vi "Tetra_TX-ATTEN_Setup.vi"() -> (0 "error out":errorcluster, 2 "Status":string="Skipping Setup of Power Supply\rDone !!!\rDONE!!\n\nSetting up PNA...\rRecalling PNA Setup:  Z:\\State Files\\TEST2.csa\rDONE!!!\rSkipping Spectrum Analyzer!!!\rSkipping Setting Up Temperature...\rSetup Complete !!!")   [LabVIEW 2018]
uses:
  <vilib>/Utility/error.llb/DialogType.ctl
  Tetra_Globals.vi
  Initialize References/Sequence Globals.vi
  Infrastructure/Test Parameter Globals_1.0.0.vi
  Initialize References/Station References Global.vi
  Infrastructure/Test Result File Name Global.vi
  <vilib>/Utility/file.llb/Read Delimited Spreadsheet (string).vi
  <vilib>/Utility/file.llb/Write Delimited Spreadsheet (string).vi
  Instruments/PNA/lib functions/Agilent ENA Series.lvlib
  Instruments/Agilent N5232A PNA-L/Labview Driver/Keysight PNA Series/Keysight PNA Series.lvlib
panel:
  in  "ess_error":errorcluster
  in  "Tab Control":T1(tab)
  in  "Setup Chip (T)":bool=TRUE
  in  "Setup Power Supply (T)":bool=TRUE
  in  "Setup PNA (T)":bool=TRUE
  in  "Kill Teraterm":bool=TRUE
  in  "Setup Gantry(t)":bool=TRUE
  in  "Setup EXA(t)":bool=TRUE
  out "Success":bool
  out "MODE":bool
  out "COM PORT":string="COM4"
  out "RevC(t)":bool
  out "RBW":string="3000"
  out "Avgs":u32=4
  out "SPAN":dbl=0.1
  out "REF_LVL":dbl=10.0
  out "PS1-1(V)":dbl=18.75
  out "PS1-1(A)":dbl=1.0
  out "PS1-2(V)":dbl=5.0
  out "PS1-2(A)":dbl=1.0
  out "Use PS1-2":bool=TRUE
  out "Use PS1-1":bool=TRUE
  out "EXA State File":string="Z:\\State Files\\State_0000.state"
  out "cmd;":string
  out "TEMP":dbl=25.0
  out "TEMP?(t)":bool
  out "RF_FREQ":dbl=20.0
  out "f_ref":dbl=10.0
  out "REF_POWER":dbl=7.5
  out "Soak Time (s)":dbl=10.0 caption="Delay Time (s)"
  out "Ant":i16
  out "Gantry-Z":dbl
  out "GET_DET":bool
  out "OUT_CAL_PATH":path=path "C:/RageATE/Automated Tests/Tetra WAM/DVT/Cal Files/OUTPUT_CAL_080321-1118.csv"
  out "HORN_CAL_PATH":path
  out "REF_CAL_PATH":path
  out "git log":string="#RageATE gitlog: commit 9dda47de5732cf8fa6a9554b7d9ab91f125b5971\n#RageATE gitlog: Author: rick-rage <rick@ragesystems.com>\n#RageATE gitlog: Date:   Mon Aug 2 15:21:18 2021 -0400\n#RageATE gitlog: This Computer Name : CRANES\r\n\r\n"
  out "PNA State File":string="Z:\\State Files\\TEST2.csa"
  out "Text":refnum<vi>
  out "OUT_CAL_PATH(str)":string
  out "Pmic_FwRev":string
  out "i_mon":string
  out "rev":string="rdiv\r\n0)  sw3p6:   195 mA  3616 mV\r\n1)  sw5p5:    89 mA  5472 mV\r\n2) sw2p8a:   315 mA  2784 mV\r\n3) sw2p8b:   349 mA  2768 mV\r\n4)  sw2p4:  1458 mA  2288 mV\r\n5)  sw1p4:  1047 mA  1304 mV\r\n>"
  out "snic":string="#Family: 0x2D\n#Serial: 0x000036092740\r\n"
  in  "error in (no error)":errorcluster
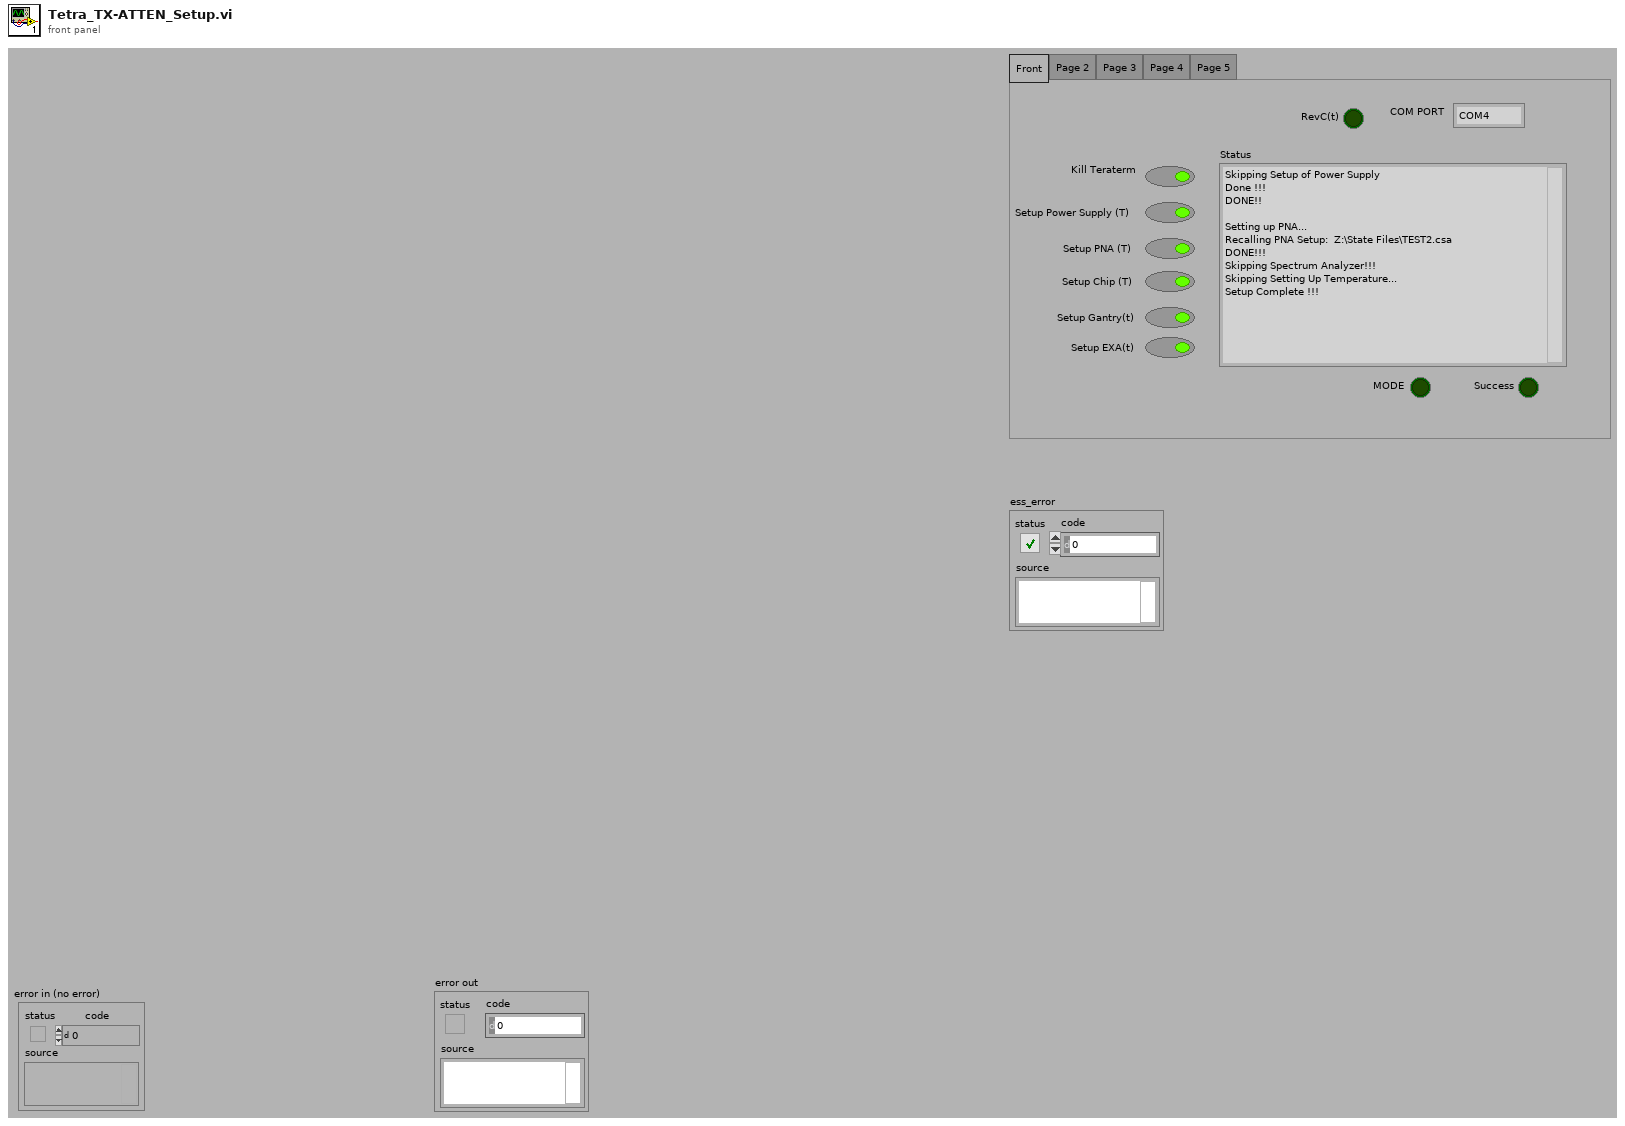
[diagram p1: front panel]
types:
  T1 = enum32{"Front", "Page 2", "Page 3", "Page 4", "Page 5"}
  T2 = typedef "DialogType.ctl" = u16
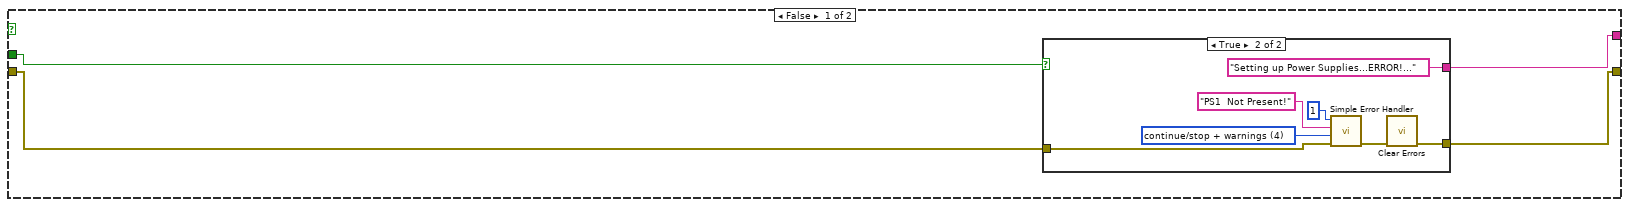
[diagram p8: hidden frame]
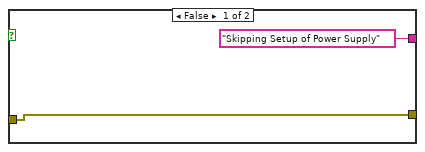
[diagram p9: hidden frame]
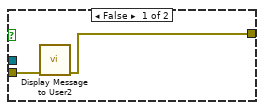
[diagram p11: hidden frame]
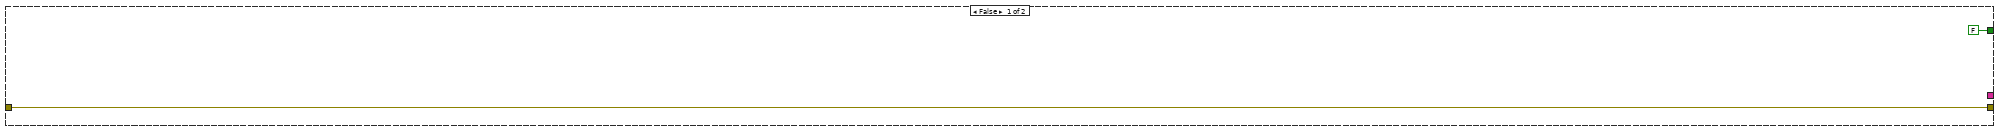
[diagram p12: hidden frame]
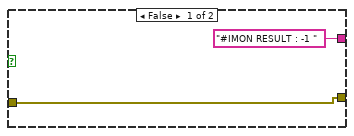
[diagram p13: hidden frame]
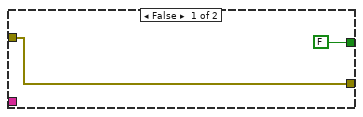
[diagram p14: hidden frame]
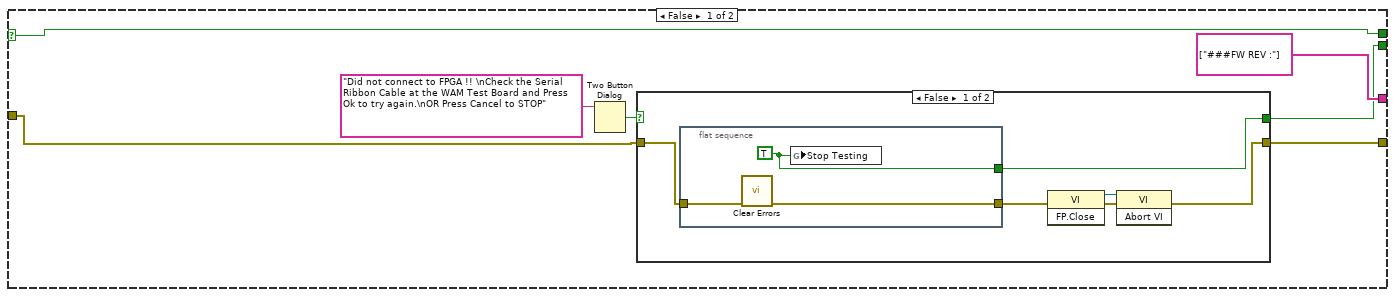
[diagram p15: hidden frame]
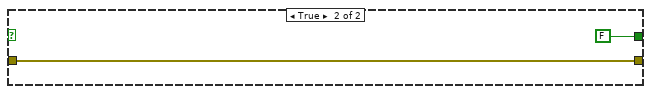
[diagram p16: hidden frame]
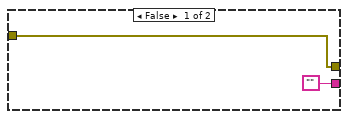
[diagram p17: hidden frame]
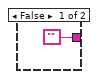
[diagram p19: hidden frame]
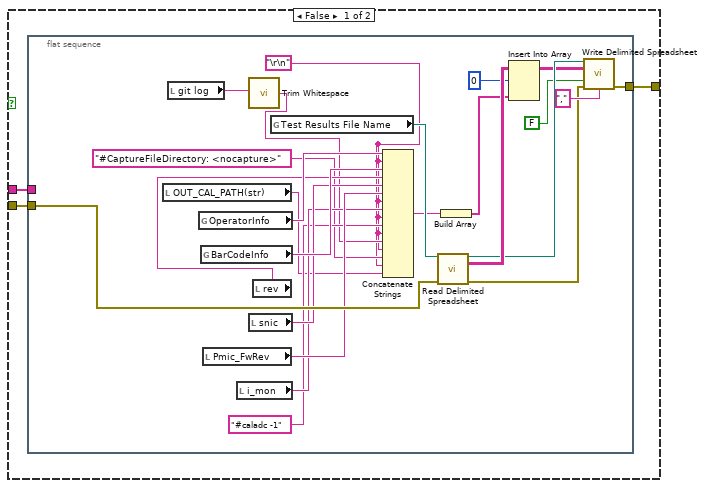
[diagram p20: hidden frame]
diagram:
  n1 = flat-sequence {
    tunnel: [w52] -> w6
    tunnel: [w51] -> w5
    tunnel: w6 -> [w111]
    tunnel: w5 -> [w110]
    tunnel: [w251] -> w8
    tunnel: [w249] -> w7
    tunnel: w8 -> [w441]
    tunnel: w7 -> [w439]
    tunnel: [w435] -> w3
    tunnel: [w520] -> w4
    tunnel: w3 -> [w523]
    tunnel: w4 -> [w591]
    tunnel: [w586] -> w10
    tunnel: [w590] -> w9
    tunnel: w10 -> [w629]
    tunnel: w9 -> [w632]
    tunnel: [w621] -> w1
    frame #0 {
      # "Automated Tests\\Tetra WAM\\PRODUCTION\\Test Benches"
      # "Kill TeraTerm"
      n2 = flat-sequence {
        tunnel: [w38] -> w16
        frame #0 {
          w35 = 1 items=["INPUT", "OUTPUT"] ("line index")
          (unwired) path "C:/RageATE/Automated Tests/Tetra WAM/PRODUCTION/Test Benches" ("base path")
          n3 = global read "Sequence Globals.vi" "DevSupportPath"() -> (w27:path)
          n4 = Strip Path(path=w27) -> (stripped path=w26:path)  [unwired: 1 out]
          n5 = global read "Sequence Globals.vi" "AppSupportPath"() -> (w32:path)
          n6 = Build Path(base path=w26, name or relative path=path "Automated Tests/Tetra WAM/PRODUCTION/Test Benches" ("base path")) -> (appended path=w24:path)
          n7 = global read "Sequence Globals.vi" "IsRuntime?"() -> (w23:bool)
          n8 = global read "Tetra_Globals.vi" "TestBench_ID"() -> (w28:string)
          n9 = Build Path(base path=w24, name or relative path=w28) -> (appended path=w37:path)
          n10 = Concatenate Strings(w28, " Calibration Files" ("name or relative path")) -> (w29:string)
          n11 = Build Path(base path=w37, name or relative path=w29) -> (appended path=w34:path)
          n12 = Select(t=w32, s=w23, f=w34) -> (s? t:f=w33:path)
          n13 = call "FindMostRecentCalFile.vi"("DIR_IN"=w33, "Test Bench (for filename match)"=w28, "line index"=w35, "IsRuntime?"=w23) -> ("Success?(t)"=w30:bool, "cal_path_out"=w31:path)  [unwired: 9 in, 1 out]
          n14 = case shown="False" w30 {
            tunnel: [path "" ("appended path") w41] -> w38
            tunnel: w31 -> [_ w41]
            frame False {
              n15 = Two Button Dialog(message="There Are No OUTPUT cal files") -> ()  [unwired: 2 in, 1 out]
            }
            frame True {
            }
          }
        }
      }
      n16 = global read "Sequence Globals.vi" "RageATE_Gitlog"() -> (→"git log":string)
      n17 = global read "Tetra_Globals.vi" "RevC(t)"() -> (→"RevC(t)":bool)
      n18 = case shown="True" "Kill Teraterm" {
        tunnel: "error in (no error)" -> [w42 w44]
        tunnel: [w42 w43] -> w18
        tunnel: "taskkill /f /im ttermpro.exe" ("command line") -> [_ w46]
        frame False {
        }
        frame True {
          n19 = call <vilib>:"Clear Errors.vi"("error in (no error)"=w44) -> ("error out"=w45:errorcluster)  [unwired: 5 in, 1 out]
          n20 = call <vilib>:"System Exec.vi"("error in (no error)"=w45, "command line"=w46) -> ("error out"=w47:errorcluster)  [unwired: 6 in, 3 out]
          n21 = call "Time Delay2"("error in (no error)"=w47) -> ("error out"=w43:errorcluster)  [unwired: 10 in]
        }
      }
      n22 = property on="Status" class="Str"(error in=w18) -> (error out=w17:errorcluster, "Text"=→"Text":refnum<vi>)  [unwired: 1 in, 1 out]
      n23 = local write "error in (no error)"(w17) -> ()
      n24 = Path To String(path=w16) -> (string=w15:string)
      n25 = Concatenate Strings("#Cal_Path: " ("string"), w15) -> (→"OUT_CAL_PATH(str)":string)
      "OUT_CAL_PATH" <- w16
    }
    frame #1 {
      # "TEMP\nPS1-1_V\nRF_FREQ_OUT\nTX_PORT\nTX_FILT\nADAR_ATT\nPSA_ATT\nREF_POWER"
      n26 = local write "Success"(FALSE ("Success")) -> ()
      n27 = local write "Setup PNA (T)"("Setup PNA (T)") -> ()
      n28 = local write "Setup EXA(t)"("Setup EXA(t)") -> ()
      n29 = local write "Setup Gantry(t)"("Setup Gantry(t)") -> ()
      n30 = local write "Setup Chip (T)"("Setup Chip (T)") -> ()
      n31 = local write "Setup Power Supply (T)"("Setup Power Supply (T)") -> ()
      n32 = global read "Test Parameter Globals_1.0.0.vi" "Input Constants Out"() -> (w52:string[])
      n33 = global read "Test Parameter Globals_1.0.0.vi" "Test Parameters"() -> (w51:string[][])
      "Status" <- ""
    }
    frame #2 {
      w107 = 0 ("disabled index (col)")
      w96 = 11  # index
      n34 = Index Array(array=w110, index (row) #1=0 ("disabled index (row)"), index (col) #1=w107, index (row) #2=7 ("disabled index (row)"), index (col) #2=w107, index (row) #3=2 ("disabled index (row)"), index (col) #3=w107) -> (element #1=w105:string, element #2=w103:string, element #3=w101:string)
      n35 = Index Array(array=w111, index #6=w96) -> (element #1=w119:string, element #2=w112:string, element #3=w73:string, element #4=w100:string, element #5=w80:string, element #6=w95:string, element #7=w81:string, element #8=w97:string, element #9=→"PNA State File":string, element #10=→"EXA State File":string, element #11=→"RBW":string, element #12=w88:string, element #13=w85:string, element #14=w83:string, element #15=w57:string, element #16=w65:string)  [unwired: 15 in]
      "cmd;" <- w81
      n36 = global write "Tetra_Globals.vi" "cmd;"(w81) -> ()
      n37 = call "StringToNumberControlWithBool.vi"("String In"=w103) -> ("Number Out"=→"REF_POWER":dbl)  [unwired: 7 in, 1 out]
      n38 = call "TempControlWithBool.vi"("INPUT"=w105) -> ("out"=→"TEMP":dbl, "Valid(t)"=→"TEMP?(t)":bool)  [unwired: 6 in, 1 out]
      n39 = call "StringToNumberControlWithBool.vi"("String In"=w101) -> ("Number Out"=w93:dbl)  [unwired: 7 in, 1 out]
      "RF_FREQ" <- w93
      n40 = global read "Tetra_Globals.vi" "comport"() -> (w71:refnum<visa-resource-name>)
      n41 = Empty String/Path?(string/path=w73) -> (empty?=w74:bool)
      n42 = global read "Sequence Globals.vi" "AppSupportPath"() -> (w68:path)
      n43 = call "StringToNumberControlWithBool.vi"("String In"=w100) -> ("NOT = 0"=→"MODE":bool)  [unwired: 7 in, 1 out]
      n44 = call "StringToNumberControlWithBool.vi"("String In"=w95) -> ("NOT = 0"=→"GET_DET":bool)  [unwired: 7 in, 1 out]
      n45 = call "StringToNumberControlWithBool.vi"("String In"=w97) -> ("Number Out"=→"Soak Time (s)":dbl)  [unwired: 7 in, 1 out]
      n46 = call "StringToNumberControlWithBool.vi"("String In"=w88) -> ("Number Out"=→"Avgs":dbl)  [unwired: 7 in, 1 out]
      n47 = call "StringToNumberControlWithBool.vi"("String In"=w85) -> ("Number Out"=→"REF_LVL":dbl)  [unwired: 7 in, 1 out]
      n48 = call "StringToNumberControlWithBool.vi"("String In"=w83) -> ("Number Out"=→"SPAN":dbl)  [unwired: 7 in, 1 out]
      n49 = global read "Sequence Globals.vi" "IsRuntime?"() -> (w70:bool)
      n50 = String To Path(string=w57) -> (path=→"REF_CAL_PATH":path)
      n51 = Divide(x=w93, y=2.0) -> (x/y=→"f_ref":dbl)
      n52 = Match Pattern(string=w119, regular expression=";") -> (before substring=w126:string, after substring=w125:string)  [unwired: 1 in, 2 out]
      n53 = Match Pattern(string=w112, regular expression=";") -> (before substring=w117:string, after substring=w116:string)  [unwired: 1 in, 2 out]
      n54 = Match Pattern(string=w80, regular expression=";") -> (before substring=w78:string, after substring=w77:string)  [unwired: 1 in, 2 out]
      n55 = Select(t=w71, s=w74, f=w73) -> (s? t:f=→"COM PORT":refnum<visa-resource-name>)
      n56 = call "StringToNumberControlWithBool.vi"("String In"=w125) -> ("Number Out"=→"PS1-1(A)":dbl)  [unwired: 7 in, 1 out]
      n57 = call "StringToNumberControlWithBool.vi"("String In"=w116) -> ("Number Out"=→"PS1-2(A)":dbl)  [unwired: 7 in, 1 out]
      n58 = call "StringToNumberControlWithBool.vi"("String In"=w126) -> ("Number Out"=→"PS1-1(V)":dbl, "NOT = 0"=→"Use PS1-1":bool)  [unwired: 7 in]
      n59 = call "StringToNumberControlWithBool.vi"("String In"=w117) -> ("Number Out"=→"PS1-2(V)":dbl, "NOT = 0"=→"Use PS1-2":bool)  [unwired: 7 in]
      n60 = call "StringToNumberControlWithBool.vi"("String In"=w78) -> ("Number Out"=→"Ant":dbl, "NOT = 0"=w86:bool)  [unwired: 7 in]
      n61 = call "StringToNumberControlWithBool.vi"("String In"=w77) -> ("Number Out"=w76:dbl)  [unwired: 7 in, 1 out]
      "Gantry-Z" <- w76
      n62 = global write "Tetra_Globals.vi" "Gantry_Z"(w76) -> ()
      n63 = String To Path(string=w65) -> (path=w69:path)
      n64 = global read "Sequence Globals.vi" "DevSupportPath"() -> (w63:path)
      n65 = local write "Setup Gantry(t)"(w86) -> ()
      n66 = Strip Path(path=w69) -> (name=w59:string)  [unwired: 1 out]
      n67 = Build Path(base path=w68, name or relative path=w59) -> (appended path=w67:path)
      n68 = Strip Path(path=w63) -> (stripped path=w62:path)  [unwired: 1 out]
      n69 = Build Path(base path=w62, name or relative path="Automated Tests\\Tetra WAM\\PRODUCTION\\Test Benches\\Common") -> (appended path=w60:path)
      n70 = Build Path(base path=w60, name or relative path=w59) -> (appended path=w58:path)
      n71 = Select(t=w67, s=w70, f=w58) -> (s? t:f=→"HORN_CAL_PATH":path)
    }
    frame #3 {
      n72 = flat-sequence {
        frame #0 {
          n73 = local read "OUT_CAL_PATH"() -> (w142:path)
          n74 = call "GetCalData.vi"("Open new file T"=TRUE, "cal file path (dialog if empty)"=w142) -> ("array out"=w141:dbl[][])  [unwired: 4 in, 5 out]
          n75 = global write "Tetra_Globals.vi" "OUT_CAL"(w141) -> ()
        }
      }
      n76 = local read "error in (no error)"() -> (w129:errorcluster)
      n77 = case shown="True" FALSE {
        frame False {
        }
        frame True {
          # "Use VNA power cal built in"
          n78 = flat-sequence {
            frame #0 {
              n79 = local read "HORN_CAL_PATH"() -> (w145:path)
              n80 = call "GetCalData.vi"("Open new file T"=TRUE, "cal file path (dialog if empty)"=w145) -> ("array out"=w144:dbl[][])  [unwired: 4 in, 5 out]
              n81 = global write "Tetra_Globals.vi" "REF_CAL"(w144) -> ()
            }
          }
        }
      }
      n82 = case shown="True" TRUE {
        tunnel: w129 -> [w132 w134]
        tunnel: [w132 w133] -> w128
        frame False {
        }
        frame True {
          # "For Horn"
          n83 = flat-sequence {
            tunnel: w134 -> [w136]
            tunnel: [w135] -> w133
            frame #0 {
              n84 = local read "HORN_CAL_PATH"() -> (w139:path)
              n85 = call "GetCalData.vi"("Open new file T"=TRUE, "error in (no error)"=w136, "cal file path (dialog if empty)"=w139) -> ("error out"=w135:errorcluster, "array out"=w138:dbl[][])  [unwired: 3 in, 4 out]
              n86 = global write "Tetra_Globals.vi" "HORN_CAL"(w138) -> ()
            }
          }
        }
      }
      n87 = local write "error in (no error)"(w128) -> ()
    }
    frame #4 {
      n88 = global read "Station References Global.vi" "RF Switch Present?"() -> (w148:bool)
      n89 = local read "error in (no error)"() -> (w147:errorcluster)
      n90 = case shown="True" w148 {
        tunnel: w147 -> [w149 w153]
        tunnel: [w149 w152] -> w146
        frame False {
        }
        frame True {
          # "Set the Switch for TX"
          n91 = global read "Station References Global.vi" "RF Switch"() -> (w154:refnum<visa-resource-name>)
          n92 = call "RfSwitch_WAM_ATE.vi"("VISA_IN"=w154, "error in"=w153, "Source"=enum16{"RFSM", "PNA"}."PNA", "T/R"=enum16{"TX", "RX"}."TX") -> ("error out"=w152:errorcluster)  [unwired: 10 in, 1 out]
        }
      }
      n93 = local write "error in (no error)"(w146) -> ()
    }
    frame #5 {
    }
    frame #6 {
      n94 = local read "Setup Power Supply (T)"() -> (w161:bool)
      n95 = global read "Station References Global.vi" "PS1 Present?"() -> (w165:bool)
      n96 = local read "error in (no error)"() -> (w157:errorcluster)
      n97 = And(x=w165, y=w161) -> (x .and. y?=w163:bool)
      n98 = case shown="True" w163 {
        tunnel: [w169 w183] -> w156
        tunnel: w157 -> [w168 w185]
        tunnel: [w167 w180] -> w162
        tunnel: w161 -> [w166 _]
        frame False {
          n99 = case shown="True" w166 {
            tunnel: [w171 w174] -> w169
            tunnel: w168 -> [w171 w173]
            tunnel: ["Skipping Setup of Power Supply" "Setting up Power Supplies...ERROR!..."] -> w167
            frame False {
            }
            frame True {
              w176 = T2 4 items=["no dialog", "OK message", "continue or stop message", "OK message + warnings", "continue/stop + warnings"] ("type of dialog (OK msg:1)")
              n100 = call <vilib>:"Simple Error Handler.vi"("error code (no error:0)"=1, "error source (\" \")"="PS1  Not Present!" ("error source (\" \")"), "type of dialog (OK msg:1)"=w176, "error in (no error)"=w173) -> ("error out"=w175:errorcluster)  [unwired: 1 in, 4 out]
              n101 = call <vilib>:"Clear Errors.vi"("error in (no error)"=w175) -> ("error out"=w174:errorcluster)  [unwired: 5 in, 1 out]
            }
          }
        }
        frame True {
          n102 = for {
            N: 2 -> [w198]
            shift-right: [w193] -> w183
            shift-left: w185 -> [w209]
            tunnel: [w189] -> w182
            tunnel: [w188] -> w181
            i -> [w200]
            stop <- w202 continue-if-true
            w191 = TRUE ("Open Ser(t)")
            n103 = stacked-sequence {
              tunnel: w209 -> [w243]
              tunnel: [w242] -> w206
              frame #0 {
                w227 = "PS1" ("SEL_PS")
                # "Conf I/V lim"
                n104 = local read "Text"() -> (w230:refnum<vi>)
                n105 = local read "PS1-1(V)"() -> (w237:dbl)
                n106 = local read "PS1-2(V)"() -> (w238:dbl)
                n107 = property class="Txt"(reference=w230, error in=w243, "Scroll Position"=i16 -1) -> (error out=w228:errorcluster)  [unwired: 1 out]
                n108 = local read "PS1-1(A)"() -> (w240:dbl)
                n109 = local read "PS1-2(A)"() -> (w239:dbl)
                n110 = global read "Station References Global.vi" "PS1"() -> (w241:refnum<visa-resource-name>)
                n111 = Build Array(w237, w238, 12.0 ("element")) -> (w232:dbl[])
                n112 = Build Array(w240, w239, 1.0 ("element")) -> (w233:dbl[])
                n113 = call "PS_SETUP_V-I-EN.vi"("VISA resource name"=w241, "SEL_PS"=w227, "error in (no error)"=w228, "Use Channel"=bool[] [FALSE, FALSE, FALSE, FALSE], "Current Lim"=w233, "Voltage Set"=w232) -> ("VISA resource name out"=w231:refnum<visa-resource-name>, "error out"=w235:errorcluster)  [unwired: 8 in]
                n114 = call "Time Delay"("error in (no error)"=w235) -> ("error out"=w226:errorcluster)  [unwired: 10 in]
                n115 = call "PS_SETUP_V-I-EN.vi"("VISA resource name"=w231, "SEL_PS"=w227, "error in (no error)"=w226, "Use Channel"=bool[] [TRUE, FALSE, FALSE, FALSE], "Current Lim"=w233, "Voltage Set"=w232) -> ("error out"=w242:errorcluster)  [unwired: 8 in, 1 out]
              }
            }
            n116 = Increment(x=w200) -> (x+1=w199:i32)
            n117 = Equal?(x=w198, y=w199) -> (x = y?=w197:bool)
            n118 = control-ref of="Text"() -> (w195:refnum<vi>)
            n119 = local read "Text"() -> (w208:refnum<vi>)
            n120 = call "BuildStrings_Return.vi"("New String"="Power Supplies ON!", "error in (no error)"=w206, "reference"=w208) -> ("error out"=w205:errorcluster, "concatenated string"=w204:string)  [unwired: 6 in, 1 out]
            n121 = local write "Status"(w204) -> ()
            n122 = control-ref of="Status"() -> (w194:refnum<vi>)
            n123 = call "DcPreBootTest.vi"("String in"=w194, "lsl/hsl limit"=dbl[] [0.01, 0.6], "reference in"=w195, "concatenated string"=w204, "error in (no error)"=w205, "seconds to wait"=2.0) -> ("DcLow?(t= low)"=w203:bool, "FlagDC?(t)"=w202:bool, "error out"=w201:errorcluster)  [unwired: 6 in, 1 out]
            n124 = global read "Station References Global.vi" "PS1"() -> (w196:refnum<visa-resource-name>)
            n125 = case shown="True" w203 {
              selector: w203 -> [_ w214]
              tunnel: w201 -> [w210 w216]
              tunnel: [w210 w215] -> w192
              tunnel: w197 -> [_ w213]
              tunnel: w196 -> [_ w211]
              frame False {
              }
              frame True {
                n126 = And(x=w214, y=w213) -> (x .and. y?=w212:bool)
                n127 = case shown="True" w212 {
                  tunnel: w216 -> [w218 w222]
                  tunnel: [w217 w219] -> w215
                  tunnel: w211 -> [_ w223]
                  frame False {
                    n128 = call "Display Message to User2"("error in (no error)"=w218) -> ("error out"=w217:errorcluster)  [unwired: 9 in, 1 out]
                  }
                  frame True {
                    n129 = call "PS_SETUP_V-I-EN.vi"("VISA resource name"=w223, "error in (no error)"=w222, "Use Channel"=bool[] [FALSE, FALSE, FALSE, FALSE]) -> ("error out"=w220:errorcluster)  [unwired: 11 in, 1 out]
                    n130 = call "Display Message to User3"("error in (no error)"=w220) -> ("error out"=w219:errorcluster)  [unwired: 9 in, 1 out]
                    n131 = invoke class="VI" method="FP.Close"(error in=w219) -> ()  [unwired: 2 in, 3 out]
                  }
                }
              }
            }
            n132 = local read "COM PORT"() -> (w190:string)
            n133 = call "Tetra Serial.vi"("COMPORT"=w190, "error in (no error)"=w192, "Open Ser(t)"=w191, "Close Ser(t)"=w191) -> ("Success"=w189:bool, "output"=w188:string, "error out"=w193:errorcluster)  [unwired: 7 in, 2 out]
          }
          n134 = local read "Status"() -> (w179:string)
          n135 = Select(t=w179, s=w182, f=w181) -> (s? t:f=w180:string)
        }
      }
      n136 = local read "Text"() -> (w158:refnum<vi>)
      n137 = call "BuildStrings_Return.vi"("seconds to wait"=0.1, "Input String"=w162, "New String"="Done !!!", "error in (no error)"=w156, "reference"=w158) -> ("error out"=w155:errorcluster, "concatenated string"=w160:string)  [unwired: 4 in, 1 out]
      n138 = local write "Status"(w160) -> ()
      n139 = local write "error in (no error)"(w155) -> ()
    }
    frame #7 {
      n140 = local read "error in (no error)"() -> (w245:errorcluster)
      n141 = local read "Setup Chip (T)"() -> (w244:bool)
      n142 = case shown="True" w244 {
        tunnel: [FALSE w263] -> w257
        tunnel: [w259 w262] -> w256
        tunnel: [_ w261] -> w253
        tunnel: w245 -> [w259 w260]
        frame False {
        }
        frame True {
          n143 = while {
            tunnel: [w288] -> w263
            tunnel: [w286] -> w261
            shift-right: [w287] -> w262
            shift-left: w260 -> [w264]
            i -> [w267]
            stop <- w270 stop-if-true
            n144 = local read "Status"() -> (w279:string)
            n145 = local read "Text"() -> (w280:refnum<vi>)
            n146 = call "BuildStrings_Return.vi"("Input String"=w279, "New String"="Booting up FPGA..." ("Delay text ..."), "error in (no error)"=w264, "reference"=w280) -> ("error out"=w273:errorcluster, "concatenated string"=w281:string)  [unwired: 5 in, 1 out]
            n147 = local write "Status"(w281) -> ()
            n148 = local read "Setup Chip (T)"() -> (w282:bool)
            n149 = call "Time Delay3"("error in (no error)"=w273, "Delay Time (s)"=10.0 ("seconds to wait")) -> ("error out"=w274:errorcluster)  [unwired: 9 in]
            n150 = local read "COM PORT"() -> (w265:string)
            n151 = case shown="True" w282 {
              tunnel: [FALSE ("Success") w314] -> w276
              tunnel: w274 -> [w300 w306]
              tunnel: [w300 w313] -> w277
              tunnel: w265 -> [_ w307]
              frame False {
              }
              frame True {
                n152 = VISA Close(VISA resource name=w307) -> (error out=w308:errorcluster)  [unwired: 1 in]
                n153 = call "Tetra Serial.vi"("COMPORT"=w307, "error in (no error)"=w308, "Command"="", "Open Ser(t)"=TRUE, "Close Ser(t)"=FALSE) -> ("Success"=w314:bool, "comport"=w310:refnum<visa-resource-name>, "error out"=w313:errorcluster)  [unwired: 6 in, 2 out]
                n154 = local read "Status"() -> (w304:string)
                n155 = global write "Tetra_Globals.vi" "comport"(w310) -> ()
                n156 = local read "Text"() -> (w305:refnum<vi>)
                n157 = call "BuildStrings_Return.vi"("Input String"=w304, "New String"="Opening Serial Port\n...Creating Global Ref", "error in (no error)"=w306, "reference"=w305) -> ("concatenated string"=w302:string)  [unwired: 5 in, 2 out]
                n158 = local write "Status"(w302) -> ()
              }
            }
            "Success" <- w276
            n159 = local read "Setup Chip (T)"() -> (w283:bool)
            n160 = And(x=w283, y=w276) -> (x .and. y?=w284:bool)
            n161 = case shown="True" w276 {
              tunnel: [w290 w299] -> w278
              tunnel: w277 -> [w290 w298]
              tunnel: ["#IMON RESULT : -1 " ("string") w292] -> w275
              frame False {
              }
              frame True {
                n162 = control-ref of="Text"() -> (w297:refnum<vi>)
                n163 = local read "COM PORT"() -> (w291:string)
                n164 = control-ref of="Status"() -> (w296:refnum<vi>)
                n165 = call <vilib>:"Trim Whitespace.vi"("string"="#IMON_RESULT: ") -> ("trimmed string"=w294:string)  [unwired: 1 in]
                n166 = call "WAM-DC-HealthCheck.vi"("COMPORT"=w291, "error in (no error)"=w298, "reference in"=w296, "LVObjectRefNum in"=w297) -> ("error out"=w299:errorcluster, "i_mon"=w293:string)  [unwired: 5 in, 1 out]
                n167 = Concatenate Strings(w294, w293) -> (w292:string)
              }
            }
            "i_mon" <- w275
            n168 = case shown="True" w284 {
              selector: w284 -> [w321 w369]
              tunnel: w278 -> [w317 w346]
              tunnel: [w316 w367] -> w287
              tunnel: [w321 w369] -> w288
              tunnel: [string[] ["###FW REV :"] ("new element/subarray") w368] -> w286
              tunnel: [w315 TRUE ("stop? (T)")] -> w271
              frame False {
                n169 = Two Button Dialog(message="Did not connect to FPGA !! \nCheck the Serial Ribbon Cable at the WAM Test Board and Press Ok to try again.\nOR Press Cancel to STOP") -> (T button?=w319:bool)  [unwired: 2 in]
                n170 = case shown="False" w319 {
                  tunnel: w317 -> [w326 w332]
                  tunnel: [w325 w332] -> w316
                  tunnel: [w327 FALSE] -> w315
                  frame False {
                    n171 = flat-sequence {
                      tunnel: [w330] -> w327
                      tunnel: w326 -> [w329]
                      tunnel: [w328] -> w323
                      frame #0 {
                        w330 = TRUE ("stop? (T)")
                        n172 = call <vilib>:"Clear Errors.vi"("error in (no error)"=w329) -> ("error out"=w328:errorcluster)  [unwired: 5 in, 1 out]
                        n173 = global write "Sequence Globals.vi" "Stop Testing"(w330) -> ()
                      }
                    }
                    n174 = invoke class="VI" method="FP.Close"(error in=w323) -> (reference out=w324:refnum<vi>, error out=w322:errorcluster)  [unwired: 2 in, 1 out]
                    n175 = invoke class="VI" method="Abort VI"(reference=w324, error in=w322) -> (error out=w325:errorcluster)  [unwired: 1 in, 2 out]
                  }
                  frame True {
                  }
                }
              }
              frame True {
                w337 = FALSE ("OpenSerial(t)")
                n176 = local read "MODE"() -> (w347:bool)
                n177 = case shown="True" w347 {
                  tunnel: ["" ";wr reg 0x04 1032;" ("string")] -> w344
                  tunnel: w346 -> [w370 w375]
                  tunnel: [w370 w374] -> w345
                  frame False {
                  }
                  frame True {
                    n178 = local read "Status"() -> (w377:string)
                    n179 = call "BuildStrings_Return.vi"("seconds to wait"=1.0, "Input String"=w377, "New String"="Setting Freq mode to Auto" ("Command"), "error in (no error)"=w375) -> ("error out"=w374:errorcluster, "concatenated string"=w373:string)  [unwired: 5 in, 1 out]
                    n180 = local write "Status"(w373) -> ()
                  }
                }
                n181 = local read "GET_DET"() -> (w357:bool)
                n182 = case shown="True" w357 {
                  tunnel: ["" "wr txm 0x49 0F" ("Command")] -> w348
                  frame False {
                  }
                  frame True {
                  }
                }
                n183 = global read "Tetra_Globals.vi" "comport"() -> (w340:refnum<visa-resource-name>)
                n184 = Concatenate Strings("seq off;" ("Command"), w348, w344) -> (w350:string)
                n185 = call "SerRW-Array.vi"("COMPORT"=w340, "error in (no error)"=w345, "Command ( ; seperation)"=w350) -> ("comport"=w342:refnum<visa-resource-name>, "error out"=w343:errorcluster)  [unwired: 6 in, 5 out]
                n186 = call "Tetra_Rev.vi"("COMPORT"=w342, "error in (no error)"=w343) -> ("rev"=w364:string, "comport"=w362:refnum<visa-resource-name>, "error out"=w361:errorcluster)  [unwired: 9 in, 2 out]
                "rev" <- w364
                n187 = global read "Tetra_Globals.vi" "BarCodeESN"() -> (w334:string)
                n188 = call "Tetra_ReadESN.vi"("COMPORT"=w362, "BC_Esn"=w334, "error in (no error)"=w361) -> ("read"=w360:string, "esn"=w358:string, "error out"=w359:errorcluster)  [unwired: 8 in, 2 out]
                "snic" <- w360
                n189 = global write "Tetra_Globals.vi" "ESN"(w358) -> ()
                n190 = local read "cmd;"() -> (w353:string)
                n191 = call "ESNLookup.vi"("ESN"=w358, "error in"=w359) -> ("error out"=w341:errorcluster)  [unwired: 7 in, 2 out]
                n192 = Empty String/Path?(string/path=w353) -> (empty?=w355:bool)
                n193 = call "UCD_Device-Info.vi"("COMPORT"=w340, "error in (no error)"=w341, "OpenSerial(t)"=w337, "CloseSerial(t)"=w337) -> ("Pmic_FwRev"=w335:string, "comport"=w339:refnum<visa-resource-name>, "error out"=w338:errorcluster)  [unwired: 8 in, 1 out]
                "Pmic_FwRev" <- w335
                n194 = case shown="False" w355 {
                  tunnel: w339 -> [w382 _]
                  tunnel: w338 -> [w381 w383]
                  tunnel: [w380 w383] -> w354
                  tunnel: w353 -> [w379 _]
                  frame False {
                    n195 = call "SerRW-Array.vi"("COMPORT"=w382, "error in (no error)"=w381, "Command ( ; seperation)"=w379) -> ("error out"=w380:errorcluster)  [unwired: 6 in, 6 out]
                  }
                  frame True {
                  }
                }
                n196 = Concatenate Strings(w364, w360, "\r\n", w335) -> (w356:string)
                n197 = Concatenate Strings("FPGA Booted : " ("string"), w364, w356) -> (w365:string)
                n198 = local read "Status"() -> (w352:string)
                n199 = local read "Text"() -> (w351:refnum<vi>)
                n200 = Build Array(w356) -> (w368:string[])
                n201 = call "BuildStrings_Return.vi"("Input String"=w352, "New String"=w365, "error in (no error)"=w354, "reference"=w351) -> ("error out"=w367:errorcluster, "concatenated string"=w366:string)  [unwired: 5 in, 1 out]
                n202 = local write "Status"(w366) -> ()
              }
            }
            n203 = Increment(x=w267) -> (x+1=w266:i32)
            n204 = Equal?(x=w266, y=2) -> (x = y?=w269:bool)
            n205 = Or(x=w271, y=w269) -> (x .or. y?=w270:bool)
          }
        }
      }
      n206 = And(x=w257, y=FALSE) -> (x .and. y?=w255:bool)
      n207 = case shown="True" w255 {
        tunnel: w256 -> [w388 w415]
        tunnel: [w387 w414] -> w252
        tunnel: w253 -> [w386 w413]
        frame False {
          n208 = flat-sequence {
            tunnel: w388 -> [w405]
            tunnel: [w404] -> w387
            tunnel: w386 -> [_]
            frame #0 {
              w390 = "\r\n"
              n209 = local read "OUT_CAL_PATH(str)"() -> (w389:string)
              n210 = local read "git log"() -> (w393:string)
              n211 = global read "Test Parameter Globals_1.0.0.vi" "OperatorInfo"() -> (w400:string)
              n212 = global read "Test Parameter Globals_1.0.0.vi" "BarCodeInfo"() -> (w399:string)
              n213 = local read "Pmic_FwRev"() -> (w396:string)
              n214 = local read "i_mon"() -> (w395:string)
              n215 = call <vilib>:"Trim Whitespace.vi"("string"=w393) -> ("trimmed string"=w392:string)  [unwired: 1 in]
              n216 = local read "snic"() -> (w397:string)
              n217 = local read "rev"() -> (w398:string)
              n218 = global read "Test Result File Name Global.vi" "Test Results File Name"() -> (w412:path)
              n219 = Concatenate Strings(w400, w390, w399, w398, w397, w396, w390, w395, w390, "#caladc -1" ("string"), w390, w392, w390, "#CaptureFileDirectory: <nocapture>" ("string"), w390, w389) -> (w402:string)
              n220 = call-poly <vilib>:"Read Delimited Spreadsheet.vi"("file path (dialog if empty)"=w412, "error in (no error)"=w405) -> ("new file path (Not A Path if cancelled)"=w410:path, "all rows"=w411:string[][], "error out"=w406:errorcluster)  [unwired: 8 in, 3 out]
              n221 = Build Array(w402) -> (w401:string[])
              n222 = Insert Into Array(array=w411, index (row)=0, new element=w401) -> (w408:string[][])  [unwired: 1 in]
              n223 = call-poly <vilib>:"Write Delimited Spreadsheet.vi"("file path (dialog if empty)"=w410, "2D data"=w408, "append to file? (new file:F)"=FALSE, "error in (no error)"=w406, "delimiter (\\t)"="," ("delimiter (\\t)")) -> ("error out"=w404:errorcluster)  [unwired: 9 in, 1 out]
            }
          }
        }
        frame True {
          n224 = flat-sequence {
            tunnel: w415 -> [w427]
            tunnel: [w426] -> w414
            tunnel: w413 -> [w424]
            frame #0 {
              n225 = global read "Test Result File Name Global.vi" "Test Results File Name"() -> (w434:path)
              n226 = global read "Test Parameter Globals_1.0.0.vi" "OperatorInfo"() -> (w419:string)
              n227 = global read "Test Parameter Globals_1.0.0.vi" "BarCodeInfo"() -> (w420:string)
              n228 = local read "git log"() -> (w423:string)
              n229 = local read "i_mon"() -> (w417:string)
              n230 = call-poly <vilib>:"Read Delimited Spreadsheet.vi"("file path (dialog if empty)"=w434, "error in (no error)"=w427) -> ("new file path (Not A Path if cancelled)"=w432:path, "all rows"=w433:string[][], "error out"=w428:errorcluster)  [unwired: 8 in, 3 out]
              n231 = Build Array(w420) -> (w421:string[])
              n232 = Build Array(w423) -> (w422:string[])
              n233 = Build Array(w419) -> (w418:string[])
              n234 = Build Array(w417) -> (w416:string[])
              n235 = Insert Into Array(array=w433, index (row)=0, new element #1=w418, new element #2=w421, new element #3=w424, new element #4=w422, new element #5=w416) -> (w430:string[][])  [unwired: 1 in]
              n236 = call-poly <vilib>:"Write Delimited Spreadsheet.vi"("file path (dialog if empty)"=w432, "2D data"=w430, "append to file? (new file:F)"=FALSE, "error in (no error)"=w428, "delimiter (\\t)"="," ("delimiter (\\t)")) -> ("error out"=w426:errorcluster)  [unwired: 9 in, 1 out]
            }
          }
        }
      }
      n237 = local read "Status"() -> (w247:string)
      n238 = local read "Text"() -> (w246:refnum<vi>)
      n239 = call "BuildStrings_Return.vi"("seconds to wait"=1.0, "Input String"=w247, "New String"="DONE!!\n\nSetting up PNA...", "error in (no error)"=w252, "reference"=w246) -> ("error out"=w251:errorcluster, "concatenated string"=w249:string)  [unwired: 4 in, 1 out]
      n240 = local write "Status"(w249) -> ()
    }
    frame #8 {
      n241 = global read "Station References Global.vi" "PNA Present?"() -> (w443:bool)
      n242 = local read "Setup PNA (T)"() -> (w444:bool)
      n243 = And(x=w444, y=w443) -> (x .and. y?=w442:bool)
      n244 = case shown="True" w442 {
        tunnel: w441 -> [w447 w490]
        tunnel: [w448 w478] -> w440
        tunnel: w439 -> [w450 w491]
        tunnel: [w446 w486] -> w438
        frame False {
          n245 = call "BuildStrings_Return.vi"("Input String"=w450, "New String"="Skipping PNA Setup...", "error in (no error)"=w447) -> ("error out"=w448:errorcluster, "concatenated string"=w446:string)  [unwired: 6 in, 1 out]
          n246 = local write "Status"(w446) -> ()
        }
        frame True {
          w460 = 0 items=["Normal", "SMC"] ("MODE")
          w459 = i64 1000000000 items=["GHz"=1000000000, "MHZ"=1000000] ("Units")
          w465 = 1 items=["Chopped", "Alternate"] ("Sweep Mode (0: Chopped)")
          w466 = 3 items=["Linear", "Logarithmic", "Power", "CW", "Segment", "Phase"] ("Sweep Type (0: Linear)")
          w481 = 1 ("Channel (1)")
          w492 = 1 items=["OFF", "ON"] ("STATE(0=OFF)")
          w494 = 3 items=["HOLD", "CONT", "GROUP", "SINGLE"]  # Mode
          w495 = 1  # Channel
          n247 = local read "PNA State File"() -> (w489:string)
          n248 = Concatenate Strings("Recalling PNA Setup:  " ("string"), w489) -> (w487:string)
          n249 = call "BuildStrings_Return.vi"("Input String"=w491, "New String"=w487, "error in (no error)"=w490) -> ("error out"=w483:errorcluster, "concatenated string"=w486:string)  [unwired: 6 in, 1 out]
          n250 = local write "Status"(w486) -> ()
          n251 = local read "Text"() -> (w485:refnum<vi>)
          n252 = property class="Txt"(reference=w485, error in=w483, "Scroll Position"=-1) -> (error out=w463:errorcluster)  [unwired: 1 out]
          n253 = for {
            N: 2 -> [_]
            tunnel: w489 -> [w505]
            tunnel: [w498] -> w454
            shift-right: [w497] -> w453
            shift-left: w463 -> [w502]
            stop <- w496 continue-if-true
            w504 = u16 0 items=["Entire Instrument State", "Segment Sweep Table", "Limit Table", "Power Sensor A", "Power Sensor B", "VBA Project", "Loss Compensation Table 1", "Loss Compensation Table 2", "Loss Compensation Table 3", "Loss Compensation Table 4", "Ripple Limit Table"] ("Data Type (0: Entire Instrument State)")
            n254 = global read "Station References Global.vi" "PNA"() -> (w500:refnum<visa-resource-name>)
            n255 = disable-structure shown="Enabled" {
              disable-tunnel: [w509 w511] -> w503
              disable-tunnel: w502 -> [w508 w511]
              disable-tunnel: [w507 w512] -> w501
              disable-tunnel: w500 -> [w506 w512]
              frame Disabled {
                n256 = call "N5232-PNA_ExecuteShortcut.vi"("Session In"=w506, "error in"=w508, "ShortcutNum"="3") -> ("Session Out"=w507:refnum<visa-resource-name>, "error out"=w509:errorcluster)  [unwired: 11 in]
              }
              frame Enabled {
              }
            }
            n257 = call "Recall.vi"("error in (no error)"=w503, "File Name ()"=w505, "Data Type (0: Entire Instrument State)"=w504, "VISA resource name"=w501) -> ("error out"=w499:errorcluster, "VISA resource name out"=w498:refnum<visa-resource-name>)  [unwired: 6 in]
            n258 = case shown="Error" w499 {
              selector: w499 -> [w513 w514]
              tunnel: w498 -> [_ w517]
              tunnel: [w513 w516] -> w497
              tunnel: [w513 w514] -> w496
              frame No Error {
              }
              frame Error {
                n259 = call <vilib>:"Clear Errors.vi"("error in (no error)"=w514) -> ("error out"=w515:errorcluster)  [unwired: 5 in, 1 out]
                n260 = call "Reset.vi"("error in (no error)"=w515, "VISA resource name"=w517) -> ("error out"=w516:errorcluster)  [unwired: 8 in, 1 out]
              }
            }
          }
          n261 = local read "f_ref"() -> (w461:dbl)
          n262 = call "PNA-L_SET-CWFREQ.vi"("Session In"=w454, "error in"=w453, "MODE"=w460, "FREQ"=w461, "Units"=w459, "CH"=1, "Source"=1) -> ("Session Out"=w455:refnum<visa-resource-name>, "error out"=w456:errorcluster)  [unwired: 10 in, 1 out]
          n263 = call "Configure Sweep.vi"("Sweep Mode (0: Chopped)"=w465, "error in (no error)"=w456, "Sweep Type (0: Linear)"=w466, "VISA resource name"=w455) -> ("error out"=w467:errorcluster, "VISA resource name out"=w468:refnum<visa-resource-name>)  [unwired: 6 in]
          n264 = call "Configure Sweep Generation.vi"("Sweep Points (201)"=1, "error in (no error)"=w467, "VISA resource name"=w468) -> ("error out"=w470:errorcluster, "VISA resource name out"=w469:refnum<visa-resource-name>)  [unwired: 7 in]
          n265 = local read "REF_POWER"() -> (w473:dbl)
          n266 = call "PNA_MAIN_RF_STATE.vi"("Session In"=w469, "error in"=w470, "RO(T)"=FALSE, "STATE(0=OFF)"=w492) -> ("Session Out"=w476:refnum<visa-resource-name>, "error out"=w475:errorcluster)  [unwired: 9 in, 1 out]
          n267 = call "Configure Power.vi"("VISA resource name"=w476, "error in (no error)"=w475, "Power Level (0 dBm)"=w473) -> ("VISA resource name out"=w477:refnum<visa-resource-name>, "error out"=w474:errorcluster)  [unwired: 11 in]
          n268 = call "PNA_SWEEP MODE.vi"("Mode"=w494, "Channel"=w495, "error in (no error)"=w474, "VISA resource name"=w477) -> ("error out"=w451:errorcluster, "VISA resource name out"=w452:refnum<visa-resource-name>)  [unwired: 6 in]
          n269 = call "Select Measurement.vi"("error in (no error)"=w451, "Measurement Name (CH1_S11_1)"="CH1_S11_1", "Channel (1)"=w481, "VISA resource name"=w452) -> ("error out"=w472:errorcluster, "VISA resource name out"=w471:refnum<visa-resource-name>)  [unwired: 6 in]
          n270 = call "Configure Marker_RageATE.vi"("Session In"=w471, "CH#"=w481, "MKR#"=1, "MKR ON(T)"=TRUE, "error in"=w472) -> ("error out"=w478:errorcluster)  [unwired: 9 in, 1 out]
        }
      }
      n271 = local read "Text"() -> (w436:refnum<vi>)
      n272 = call "BuildStrings_Return.vi"("Input String"=w438, "New String"="DONE!!!", "error in (no error)"=w440, "reference"=w436) -> ("error out"=w435:errorcluster, "concatenated string"=w437:string)  [unwired: 5 in, 1 out]
      n273 = local write "Status"(w437) -> ()
    }
    frame #9 {
      n274 = global read "Station References Global.vi" "Spectrum Analyzer Present?"() -> (w524:bool)
      n275 = local read "Setup EXA(t)"() -> (w521:bool)
      n276 = And(x=w524, y=w521) -> (x .and. y?=w522:bool)
      n277 = local read "Status"() -> (w519:string)
      n278 = case shown="True" w522 {
        tunnel: w523 -> [w528 w576]
        tunnel: [w529 w558] -> w520
        tunnel: [w525 w552] -> w518
        tunnel: w519 -> [w526 w553]
        frame False {
          n279 = local read "Text"() -> (w527:refnum<vi>)
          n280 = call "BuildStrings_Return.vi"("Input String"=w526, "New String"="Skipping Spectrum Analyzer!!!", "error in (no error)"=w528, "reference"=w527) -> ("error out"=w529:errorcluster, "concatenated string"=w525:string)  [unwired: 5 in, 1 out]
        }
        frame True {
          w556 = u16 0 items=["OFF", "ON"] ("ON/OFF")
          w566 = u16 2 items=["Hz", "MHz", "GHz"] ("Freq Units")
          w569 = 1 items=["Clear Write", "Average", "Maximum Hold", "Minimum Hold"] ("Trace Type (0: Clear Write)")
          w570 = 0 items=["RBW AUTO OFF", "RBW AUTO ON"] ("RBW AUTO")
          n281 = global read "Station References Global.vi" "Spectrum Analyzer Model"() -> (w540:string)
          n282 = global read "Station References Global.vi" "Spectrum Analyzer"() -> (w548:refnum<visa-resource-name>)
          n283 = local read "Text"() -> (w554:refnum<vi>)
          n284 = Equal?(x=w540, y="E4447A") -> (x = y?=w538:bool)
          n285 = local read "EXA State File"() -> (w561:string)
          n286 = call "BuildStrings_Return.vi"("Input String"=w553, "New String"="Setting Up Spectrum Analyzer!!!", "error in (no error)"=w576, "reference"=w554) -> ("error out"=w551:errorcluster, "concatenated string"=w552:string)  [unwired: 5 in, 1 out]
          n287 = Empty String/Path?(string/path=w561) -> (empty?=w562:bool)
          n288 = call "Instrument Mode.vi"("SKIP(T)"=w538, "SET/GET"="SET", "error in"=w551, "Select INST"="INST SA", "Session In"=w548) -> ("error out"=w550:errorcluster, "Session Out"=w549:refnum<visa-resource-name>)  [unwired: 4 in, 1 out]
          n289 = case shown="True" w562 {
            tunnel: w549 -> [w582 w584]
            tunnel: w561 -> [w581 _]
            tunnel: w550 -> [w580 w583]
            tunnel: [w579 w583] -> w568
            tunnel: [w578 w584] -> w567
            frame False {
              n290 = call "EXA_RCL_STATE.vi"("FileName"=w581, "error in"=w580, "Session In"=w582) -> ("error out"=w579:errorcluster, "Session Out"=w578:refnum<visa-resource-name>)  [unwired: 7 in]
            }
            frame True {
            }
          }
          n291 = local read "RF_FREQ"() -> (w565:dbl)
          n292 = local read "SPAN"() -> (w563:dbl)
          n293 = call "SA_SET_CF.vi"("Send OPC? (T)"=TRUE, "error in"=w568, "Freq Units"=w566, "SET CF ()"=w565, "Session In"=w567) -> ("error out"=w536:errorcluster, "Session Out"=w537:refnum<visa-resource-name>)  [unwired: 4 in, 1 out]
          n294 = call "FREQ_SPAN.vi"("error in"=w536, "Span(MHz)"=w563, "Session In"=w537) -> ("error out"=w534:errorcluster, "Session Out"=w535:refnum<visa-resource-name>)  [unwired: 6 in, 1 out]
          n295 = local read "Avgs"() -> (w573:u32)
          n296 = call "SA_AVG.vi"("Session In"=w535, "AVG Count"=w573, "error in"=w534, "Trace Type (0: Clear Write)"=w569, "AVG Restart (T)"=FALSE, "Send OPC? (T)"=FALSE) -> ("Session Out"=w575:refnum<visa-resource-name>, "error out"=w574:errorcluster)  [unwired: 8 in]
          n297 = local read "RBW"() -> (w572:string)
          n298 = local read "REF_LVL"() -> (w564:dbl)
          n299 = call "SA_RBW.vi"("Session In"=w575, "RBW(Hz)"=w572, "error in"=w574, "RO (T)"=FALSE, "RBW AUTO"=w570) -> ("Session Out"=w532:refnum<visa-resource-name>, "error out"=w533:errorcluster)  [unwired: 6 in, 3 out]
          n300 = call "REF_LEV.vi"("Session In"=w532, "RefLvl"=w564, "error in"=w533) -> ("Session Out"=w545:refnum<visa-resource-name>, "error out"=w542:errorcluster)  [unwired: 9 in, 2 out]
          n301 = call "SA_ATT.vi"("Session In"=w545, "ATT"=0.0, "error in"=w542) -> ("Session Out"=w544:refnum<visa-resource-name>, "error out"=w543:errorcluster)  [unwired: 9 in, 2 out]
          n302 = call "SWEEP_CONT.vi"("Session In"=w544, "OPC?"=TRUE, "ON/OFF"=w556, "error in"=w543, "RO (T)"=FALSE) -> ("error out"=w558:errorcluster)  [unwired: 8 in, 2 out]
        }
      }
      n303 = local write "Status"(w518) -> ()
    }
    frame #10 {
      n304 = global read "Station References Global.vi" "Oven Present?"() -> (w589:bool)
      n305 = local read "TEMP?(t)"() -> (w587:bool)
      n306 = And(x=w587, y=w589) -> (x .and. y?=w588:bool)
      n307 = local read "Status"() -> (w585:string)
      n308 = case shown="False" w588 {
        tunnel: w591 -> [w599 w619]
        tunnel: w585 -> [w597 w618]
        tunnel: [w593 w612] -> w590
        tunnel: w587 -> [w598 _]
        tunnel: [w595 w609] -> w586
        frame False {
          n309 = call "Display Message to User"("error in (no error)"=w599, "Enable"=w598) -> ("error out"=w594:errorcluster, "Cancel"=w596:bool)  [unwired: 8 in]
          n310 = global write "Station References Global.vi" "Oven Present?"(FALSE ("Oven Present?")) -> ()
          n311 = Stop(stop? (T)=w596) -> ()
          n312 = case shown="False" w596 {
            tunnel: w597 -> [w604 w607]
            tunnel: [w603 w607] -> w593
            tunnel: [w602 w606] -> w595
            tunnel: w594 -> [w601 w606]
            frame False {
              n313 = local read "Text"() -> (w600:refnum<vi>)
              n314 = call "BuildStrings_Return.vi"("Input String"=w604, "New String"="Skipping Setting Up Temperature...", "error in (no error)"=w601, "reference"=w600) -> ("error out"=w602:errorcluster, "concatenated string"=w603:string)  [unwired: 5 in, 1 out]
            }
            frame True {
            }
          }
          n315 = local write "Status"(w593) -> ()
        }
        frame True {
          n316 = local read "Text"() -> (w608:refnum<vi>)
          n317 = call "BuildStrings_Return.vi"("Input String"=w618, "New String"="Setting Up Temperature...", "error in (no error)"=w619, "reference"=w608) -> ("error out"=w616:errorcluster, "concatenated string"=w612:string)  [unwired: 5 in, 1 out]
          n318 = local write "Status"(w612) -> ()
          n319 = global read "Station References Global.vi" "Oven"() -> (w617:refnum<visa-resource-name>)
          n320 = local read "TEMP"() -> (w615:dbl)
          n321 = call "PM9 Set Temp and Wait.vi"("VISA"=w617, "Error In"=w616, "Accuracy +/-"=2.0, "Set Point"=w615, "RO(t)"=FALSE, "Min (-1 for cont.)"=0.1 ("Min"), "close session(t)"=TRUE) -> ("error out"=w609:errorcluster)  [unwired: 9 in, 3 out]
        }
      }
    }
    frame #11 {
      n322 = global read "Station References Global.vi" "Gantry Present?"() -> (w624:bool)
      n323 = local read "Setup Gantry(t)"() -> (w626:bool)
      n324 = local read "Text"() -> (w628:refnum<vi>)
      n325 = And(x=w626, y=w624) -> (x .and. y?=w625:bool)
      n326 = case shown="True" w625 {
        tunnel: "ess_error" -> [w634 w638]
        tunnel: [w634 w645] -> w623
        frame False {
        }
        frame True {
          w640 = 21.0  # z ref
          w641 = u16 0 items=["Inches", "cm"] ("Zunits")
          n327 = global read "Station References Global.vi" "Gantry"() -> (w639:refnum<visa-resource-name>)
          n328 = for {
            N: 2 -> [_]
            tunnel: w639 -> [w655]
            shift-right: [w650] -> w637
            shift-left: w638 -> [w654]
            tunnel: [w647] -> w635
            stop <- w648 stop-if-true
            w653 = TRUE ("Open Serial")
            n329 = call "WAM_ESS.vi"("VISA resource name"=w655, "error in (no error)"=w654, "Open Serial"=w653, "Test Running (T)"=w653, "Close Serial"=w653) -> ("Enabled(T-RO)"=w652:bool, "FH_NOT(T)"=w651:bool, "VISA resource name out"=w646:refnum<visa-resource-name>, "error out"=w649:errorcluster)  [unwired: 7 in]
            n330 = And(x=w652, y=w651) -> (x .and. y?=w648:bool)
            n331 = case shown="False" w648 {
              tunnel: [w664 w666] -> w650
              tunnel: w649 -> [w662 w666]
              tunnel: [w659 w665] -> w647
              tunnel: w646 -> [w658 w665]
              frame False {
                w656 = TRUE ("Close Serial")
                w657 = u16 1 items=["Disable Driver", "Enable Driver", "Read Driver Status"] ("Driver-Func")
                n332 = call "Prompt User for Input"("error in (no error)"=w662) -> ("RESET"=w661:bool, "error out"=w663:errorcluster)  [unwired: 17 in]
                n333 = Not(x=w661) -> (.not. x?=w660:bool)
                n334 = Stop(stop? (T)=w660) -> ()
                n335 = call "Gantry_Driver.vi"("VISA resource name"=w658, "error in (no error)"=w663, "Open Serial"=w656, "Driver-Func"=w657, "Close Serial"=w656) -> ("VISA resource name out"=w659:refnum<visa-resource-name>, "error out"=w664:errorcluster)  [unwired: 11 in, 2 out]
              }
              frame True {
              }
            }
          }
          n336 = local read "Gantry-Z"() -> (w642:dbl)
          n337 = local read "Ant"() -> (w643:i16)
          n338 = call "Gantry.vi"("COMPORT"=w635, "error in (no error)"=w637, "Antenna Select"=w643, "z ref"=w640, "Write(reads antenna co-ords when off)"=TRUE, "z"=w642, "Zunits"=w641) -> ("error out"=w645:errorcluster)  [unwired: 12 in]
        }
      }
      n339 = call "BuildStrings_Return.vi"("seconds to wait"=1.0, "Input String"=w632, "New String"="Setup Complete !!!", "error in (no error)"=w629, "reference"=w628) -> ("error out"=w627:errorcluster, "concatenated string"=w633:string)  [unwired: 4 in, 1 out]
      "error out" <- w627
      n340 = local write "Status"(w633) -> ()
      n341 = local write "ess_error"(w623) -> ()
      n342 = Merge Errors(w627, w623) -> (w621:errorcluster)
      n343 = global write "Test Parameter Globals_1.0.0.vi" "Setup.vi Error"(w621) -> ()
    }
  }
  n344 = Unbundle By Name(w1) -> ("source"=w2:string)  [unwired: 2 out]
  n345 = case shown="Error" w1 {
    tunnel: w2 -> [_ w667]
    frame No Error {
    }
    frame Error {
      n346 = call "Display Message to User4"("Message"=w667) -> ()  [unwired: 9 in, 2 out]
    }
  }
